vi "sub_hstr-str.vi"(11 "h-str":string="¥Z\u0003\u0000\u0000\u0000\u0006\u0000\u0000\u0000") -> (3 "h2n-str":string)   [LabVIEW 2019]
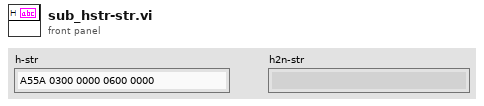
[diagram p1: front panel]
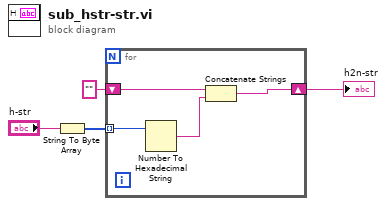
[diagram p0: block diagram]
diagram:
  n1 = String To Byte Array(string="h-str") -> (unsigned byte array=w3:u8[])
  n2 = for {
    tunnel: w3 -> [w8] mode=indexing
    shift-right: [w5] -> w1
    shift-left: "" -> [w6]
    n3 = Number To Hexadecimal String(2:w8) -> (0:w7:string)  [unwired: 1 in]
    n4 = Concatenate Strings(w6, w7) -> (w5:string)
  }
  "h2n-str" <- w1
